vi "Out.vi"(8 "error in (no error)":errorcluster, 11 "FlipMir in":refnum<class "FlipMir.lvclass">) -> (0 "error out":errorcluster, 3 "FlipMir out":refnum<class "FlipMir.lvclass">)   [LabVIEW 2016, in "FlipMir.lvclass"]
uses:
  FlipMir.lvclass
  FlipMir.lvclass/FlipMir.ctl
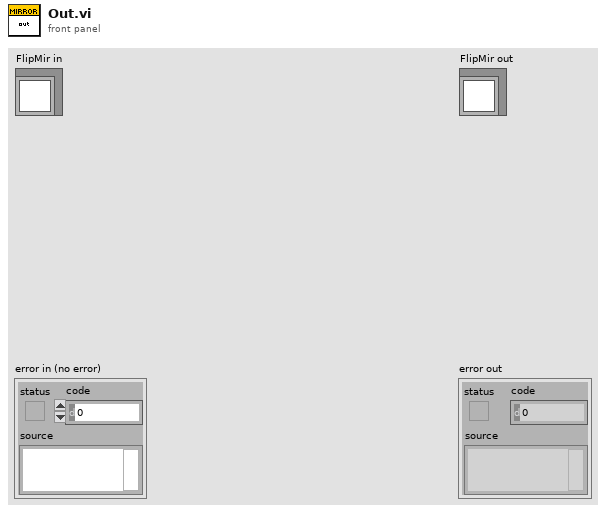
[diagram p1: front panel]
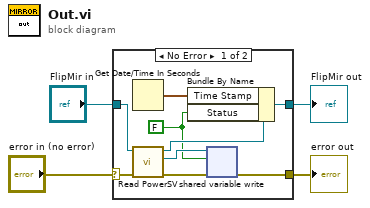
[diagram p0: block diagram]
diagram:
  n1 = case shown="No Error" "error in (no error)" {
    selector: "error in (no error)" -> [w12 w15]
    tunnel: [w5 w15] -> w3
    tunnel: [w6 w14] -> w1
    tunnel: "FlipMir in" -> [w13 w14]
    frame No Error {
      w8 = FALSE ("data in")
      n2 = Get Date/Time In Seconds() -> (seconds since 1Jan1904=w7:timestamp)
      n3 = call-dynamic "Read PowerSV.vi"("error in (no error)"=w12, "FlipMir in"=w13) -> ("error out"=w10:errorcluster, "PowerSV"=w11:refnum<k21>, "FlipMir out"=w9:refnum<class "FlipMir.lvclass">)  [unwired: 7 in]
      n4 = Bundle By Name(cluster=w9, "Time Stamp"=w7, "Status"=w8) -> (w6:refnum<class "FlipMir.lvclass">)
      n5 = shared-variable-write(w11, w10, w8) -> (w5:errorcluster)  [unwired: 1 out]
    }
    frame Error {
    }
  }
  "error out" <- w3
  "FlipMir out" <- w1
